vi "DataTreeCtrl setFileTreeMenu.vi"(8 "error in (no error)":errorcluster, 10 "menuRefnum":refnum<k9>, 11 "fileTreeRefnum":refnum<vi>) -> (0 "error out":errorcluster)   [LabVIEW 2018, in "DataTreeCtrl.lvclass"]
uses:
  DataTreeCtrl.lvclass
  ctl/menuState.ctl
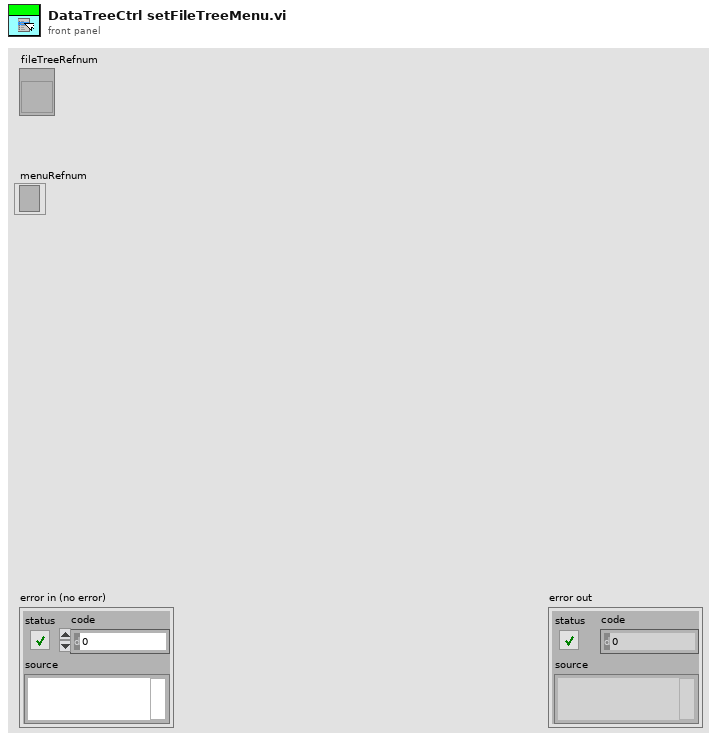
[diagram p1: front panel]
types:
  T1 = typedef "menuState.ctl" = enum16{"selectNone", "selectSingleFile", "selectSingleData", "selectMultipleDataOfSame", "selectMultipleDataOfDiff"}
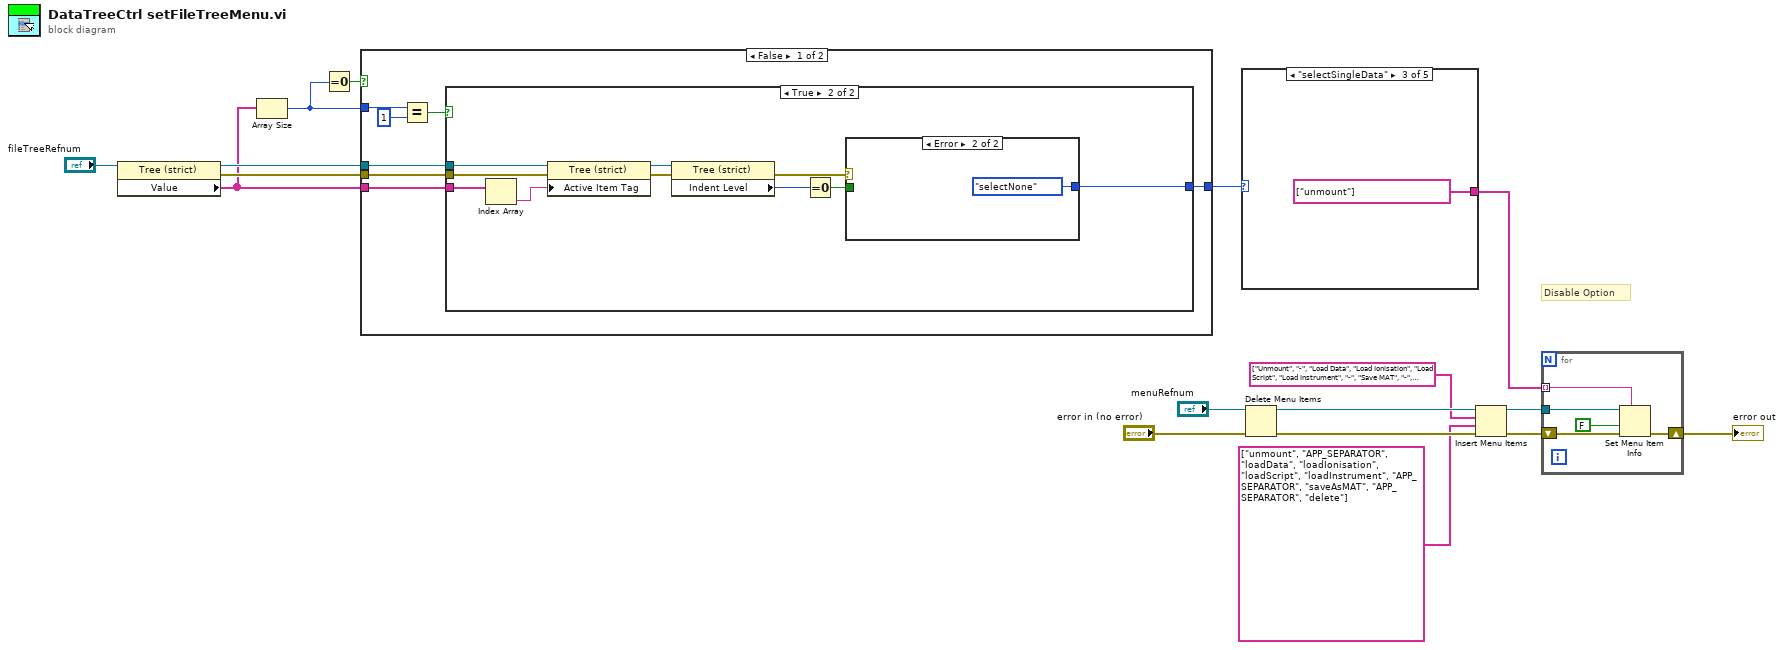
[diagram p0: block diagram]
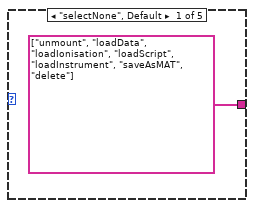
[diagram p2: hidden frame]
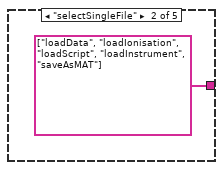
[diagram p3: hidden frame]
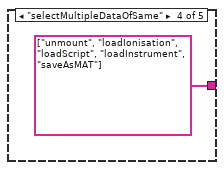
[diagram p4: hidden frame]
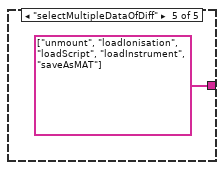
[diagram p5: hidden frame]
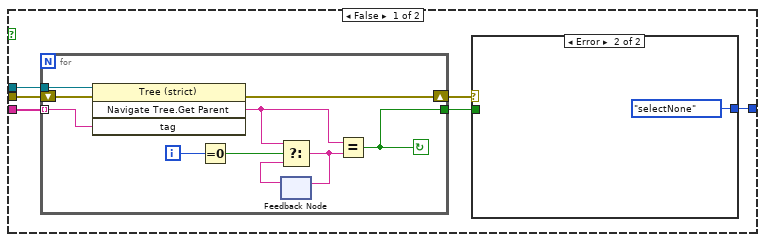
[diagram p6: hidden frame]
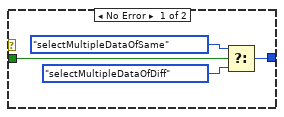
[diagram p7: hidden frame]
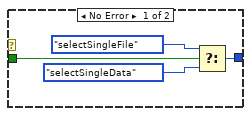
[diagram p8: hidden frame]
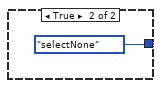
[diagram p9: hidden frame]
diagram:
  # "Disable Option"
  n1 = property class="Tree (strict)"(reference="fileTreeRefnum") -> (reference out=w12:refnum<vi>, error out=w11:errorcluster, "Value"=w10:string[])  [unwired: 1 in]
  n2 = Array Size(array=w10) -> (size(s)=w9:i32)
  n3 = Equal To 0?(x=w9) -> (x = 0?=w8:bool)
  n4 = case shown="False" w8 {
    tunnel: w12 -> [w24 _]
    tunnel: w11 -> [w23 _]
    tunnel: w10 -> [w22 _]
    tunnel: w9 -> [w21 _]
    tunnel: [w18 menuState."selectNone"] -> w7
    frame False {
      n5 = Equal?(x=w21, y=1) -> (x = y?=w19:bool)
      n6 = case shown="True" w19 {
        tunnel: w24 -> [w29 w55]
        tunnel: w23 -> [w28 w54]
        tunnel: w22 -> [w30 w53]
        tunnel: [w26 w47] -> w18
        frame False {
          n7 = for {
            tunnel: w30 -> [w43] mode=indexing
            tunnel: w29 -> [w45]
            tunnel: [w37] -> w27
            shift-right: [w36] -> w25
            shift-left: w28 -> [w44]
            i -> [w42]
            stop <- w37 continue-if-true
            n8 = invoke class="Tree (strict)" method="Navigate Tree.Get Parent"(reference=w45, error in=w44, "tag"=w43) -> (error out=w36:errorcluster, "Navigate Tree:Get Parent"=w39:string)  [unwired: 1 in, 2 out]
            n9 = Equal To 0?(x=w42) -> (x = 0?=w41:bool)
            n10 = feedback #1() -> (w40:string)  [unwired: 1 in]
            n11 = Select(t=w39, s=w41, f=w40) -> (s? t:f=w38:string)
            n12 = feedback-in #1(w38) -> ()
            n13 = Equal?(x=w39, y=w38) -> (x = y?=w37:bool)
          }
          n14 = case shown="Error" w25 {
            tunnel: w27 -> [w34 _]
            tunnel: [w31 menuState."selectNone"] -> w26
            frame No Error {
              n15 = Select(t=menuState."selectMultipleDataOfSame", s=w34, f=menuState."selectMultipleDataOfDiff") -> (s? t:f=w31:T1)
            }
            frame Error {
            }
          }
        }
        frame True {
          n16 = Index Array(array=w53) -> (element=w52:string)  [unwired: 1 in]
          n17 = property class="Tree (strict)"(reference=w55, error in=w54, "Active Item Tag"=w52) -> (reference out=w51:refnum<vi>, error out=w50:errorcluster)
          n18 = property class="Tree (strict)"(reference=w51, error in=w50) -> (error out=w46:errorcluster, "Indent Level"=w49:i32)  [unwired: 1 out]
          n19 = Equal To 0?(x=w49) -> (x = 0?=w48:bool)
          n20 = case shown="Error" w46 {
            tunnel: w48 -> [w59 _]
            tunnel: [w56 menuState."selectNone"] -> w47
            frame No Error {
              n21 = Select(t=menuState."selectSingleFile", s=w59, f=menuState."selectSingleData") -> (s? t:f=w56:T1)
            }
            frame Error {
            }
          }
        }
      }
    }
    frame True {
    }
  }
  n22 = case shown="\"selectSingleData\"" w7 {
    tunnel: [string[] ["unmount", "loadData", "loadIonisation", "loadScript", "loadInstrument", "saveAsMAT", "delete"] ("item tags") string[] ["loadData", "loadIonisation", "loadScript", "loadInstrument", "saveAsMAT"] string[] ["unmount"] string[] ["unmount", "loadIonisation", "loadScript", "loadInstrument", "saveAsMAT"] string[] ["unmount", "loadIonisation", "loadScript", "loadInstrument", "saveAsMAT"]] -> w5
    frame "selectNone", Default {
    }
    frame "selectSingleFile" {
    }
    frame "selectSingleData" {
    }
    frame "selectMultipleDataOfSame" {
    }
    frame "selectMultipleDataOfDiff" {
    }
  }
  n23 = Delete Menu Items(6:"error in (no error)", 9:"menuRefnum") -> (0:w16:errorcluster, 3:w17:refnum<k9>)  [unwired: 2 in]
  n24 = Insert Menu Items(6:w16, 7:string[] ["unmount", "APP_SEPARATOR", "loadData", "loadIonisation", "loadScript", "loadInstrument", "APP_SEPARATOR", "saveAsMAT", "APP_SEPARATOR", "delete"] ("item tags"), 8:string[] ["Unmount", "-", "Load Data", "Load Ionisation", "Load Script", "Load Instrument", "-", "Save MAT", "-", "Delete"] ("item tags"), 9:w17) -> (0:w4:errorcluster, 3:w2:refnum<k9>)  [unwired: 2 in, 1 out]
  n25 = for {
    tunnel: w5 -> [w71] mode=indexing
    shift-right: [w68] -> w3
    shift-left: w4 -> [w69]
    tunnel: w2 -> [w67]
    n26 = Set Menu Item Info(7:w71, 8:w69, 9:FALSE ("enabled"), 11:w67) -> (0:w68:errorcluster)  [unwired: 3 in, 1 out]
  }
  "error out" <- w3
